vi "IMAQdx_grab_att.vi"() -> ()   [LabVIEW 2015]
doc: "The Grab VI acquires images continuously and displays the images in an image control using low-level acquisition VIs. A grab is appropriate for high-speed applications in which you need to process only one image at a time."
uses:
  <vilib>/vision/driver/IMAQdx.llb/IMAQdx Acquisition Mode.ctl
  <vilib>/vision/driver/IMAQdx.llb/IMAQdx Buffer Number Mode.ctl
  <vilib>/vision/driver/NI_Vision_Acquisition_Software.lvlib
  <resource>/objmgr/imaqdx.rc
  <vilib>/vision/NI_Vision_Development_Module.lvlib
panel:
  out "Luminance Plane":T1(plugin-control)
  out "Image":T1(plugin-control)
  out "ValueDBL 4":dbl
  out "MinDBL 5":dbl
  out "MaxDBL 5":dbl
  out "ActVal:Gain":string
  out "ValueU32 4":u32
  out "ValueDBL 3":dbl
  out "MinDBL 4":dbl
  out "MaxDBL 4":dbl
  out "ActGainMode":string
  out "ValueU32 3":u32
  out "ValueDBL 2":dbl
  out "MinDBL 3":dbl
  out "MaxDBL 3":dbl
  out "ActValue:Exposure":string
  out "ValueU32 2":u32
  out "ValueU32":u32
  out "ActExpMode":string
  out "MaxDBL 2":dbl
  out "MinDBL 2":dbl
  out "ValueDBL":dbl
  in  "Stop 4":bool
  out "Streaming Started":bool
  out "Stream completed":bool
  in  "Set: Exposure::Value":dbl=0.0625 caption="Exposure::Value" min=0.0 max=0.125
  in  "Gain::Mode":u32(ring)=2 caption="Exposure::Mode" items=["Auto"=1, "Manual"=2]
  in  "Exposure::Mode":u32(ring)=2 items=["Auto"=1, "Manual"=2]
  in  "Set Gain":bool
  in  "Set Exposure":bool
  in  "Stop 3":bool
  out "output cluster":cluster{sgl, sgl}
  out "Last Mouse Position:All Elements":cluster{"X":i32, "Y":i32}
  in  "Set: Gain::Value":i64 caption="Gain::Value" min=0 max=1728 step=1
  in  "Pixel Distances":T2={"X Step"=5.2, "Y Step"=5.2, "Unit"=enum."Micrometer"} {"Y Step" format="%.2f"; "X Step" format="%.2f"}
  out "error out":errorcluster
  in  "Camera Name":refnum<k21>="cam0" caption="IMAQdx Session"
  out "Buffer Number":u32
  out "Frame Rate":dbl(knob) scale=0.0..20.0
  in  "Stop":bool
  # "Overview: Demonstrates how to acquire continuous images from a camera using low level acquisition functions.\nRequirements: Vision Acquisition Software\nInstructions:\n1. Select the Camera Name\n2. Run the VI"
  # "x /µm"
  # "y /µm"
  # "ExpMode"
  # "ExpVal"
  # "GainMode"
  # "GainValue"
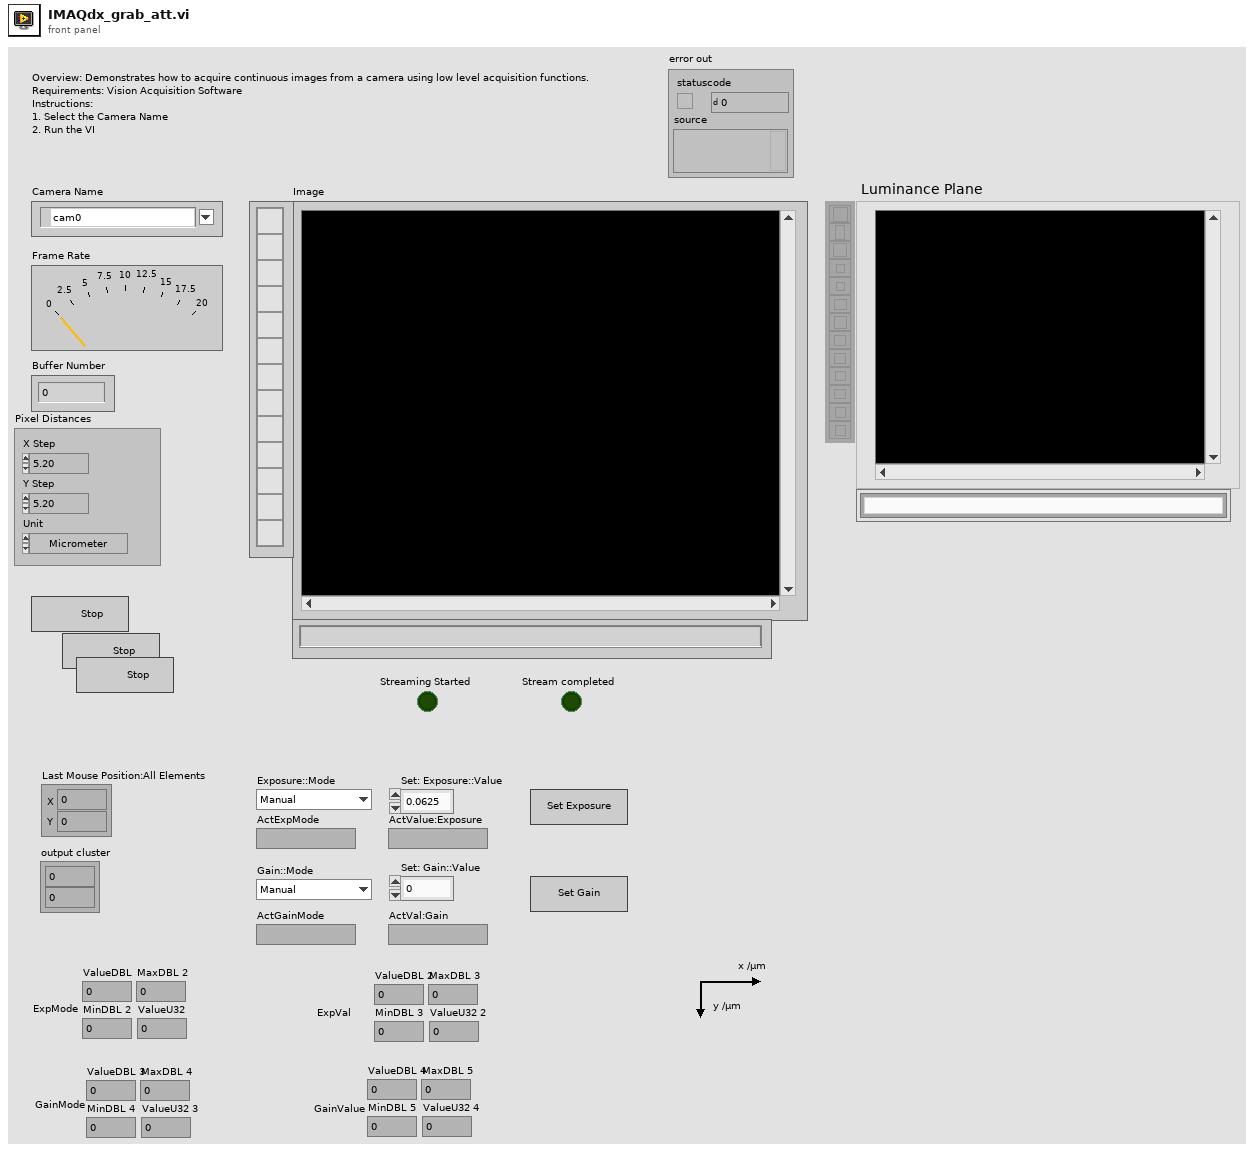
[diagram p1: front panel]
types:
  T1 = typedef "IMAQ Image.ctl" = refnum<image>
  T2 = typedef "Simple Grid Descriptor" = cluster{"X Step":sgl, "Y Step":sgl, "Unit":T3}
  T3 = typedef "Image Unit" = enum32{"Undefined", "Angström", "Micrometer", "Millimeter", "Centimeter", "Meter", "Kilometer", "Microinch", "Inch", "Feet", "Nautical miles", "Standard miles", "Steps"}
  T4 = typedef "Image Type" = u32
  T5 = typedef "NI_Vision_Acquisition_Software.lvlib/IMAQdx Acquisition Mode.ctl" = enum32{"One Shot", "Continuous"}
  T6 = typedef "IMAQdx.ctl" = refnum<k21>
  T7 = enum8{"Enabled", "Disabled", "Disabled and Grayed Out"}
  T8 = typedef "NI_Vision_Acquisition_Software.lvlib/IMAQdx Buffer Number Mode.ctl" = enum32{"Next", "Last", "Buffer Number", "Every", "Last New"}
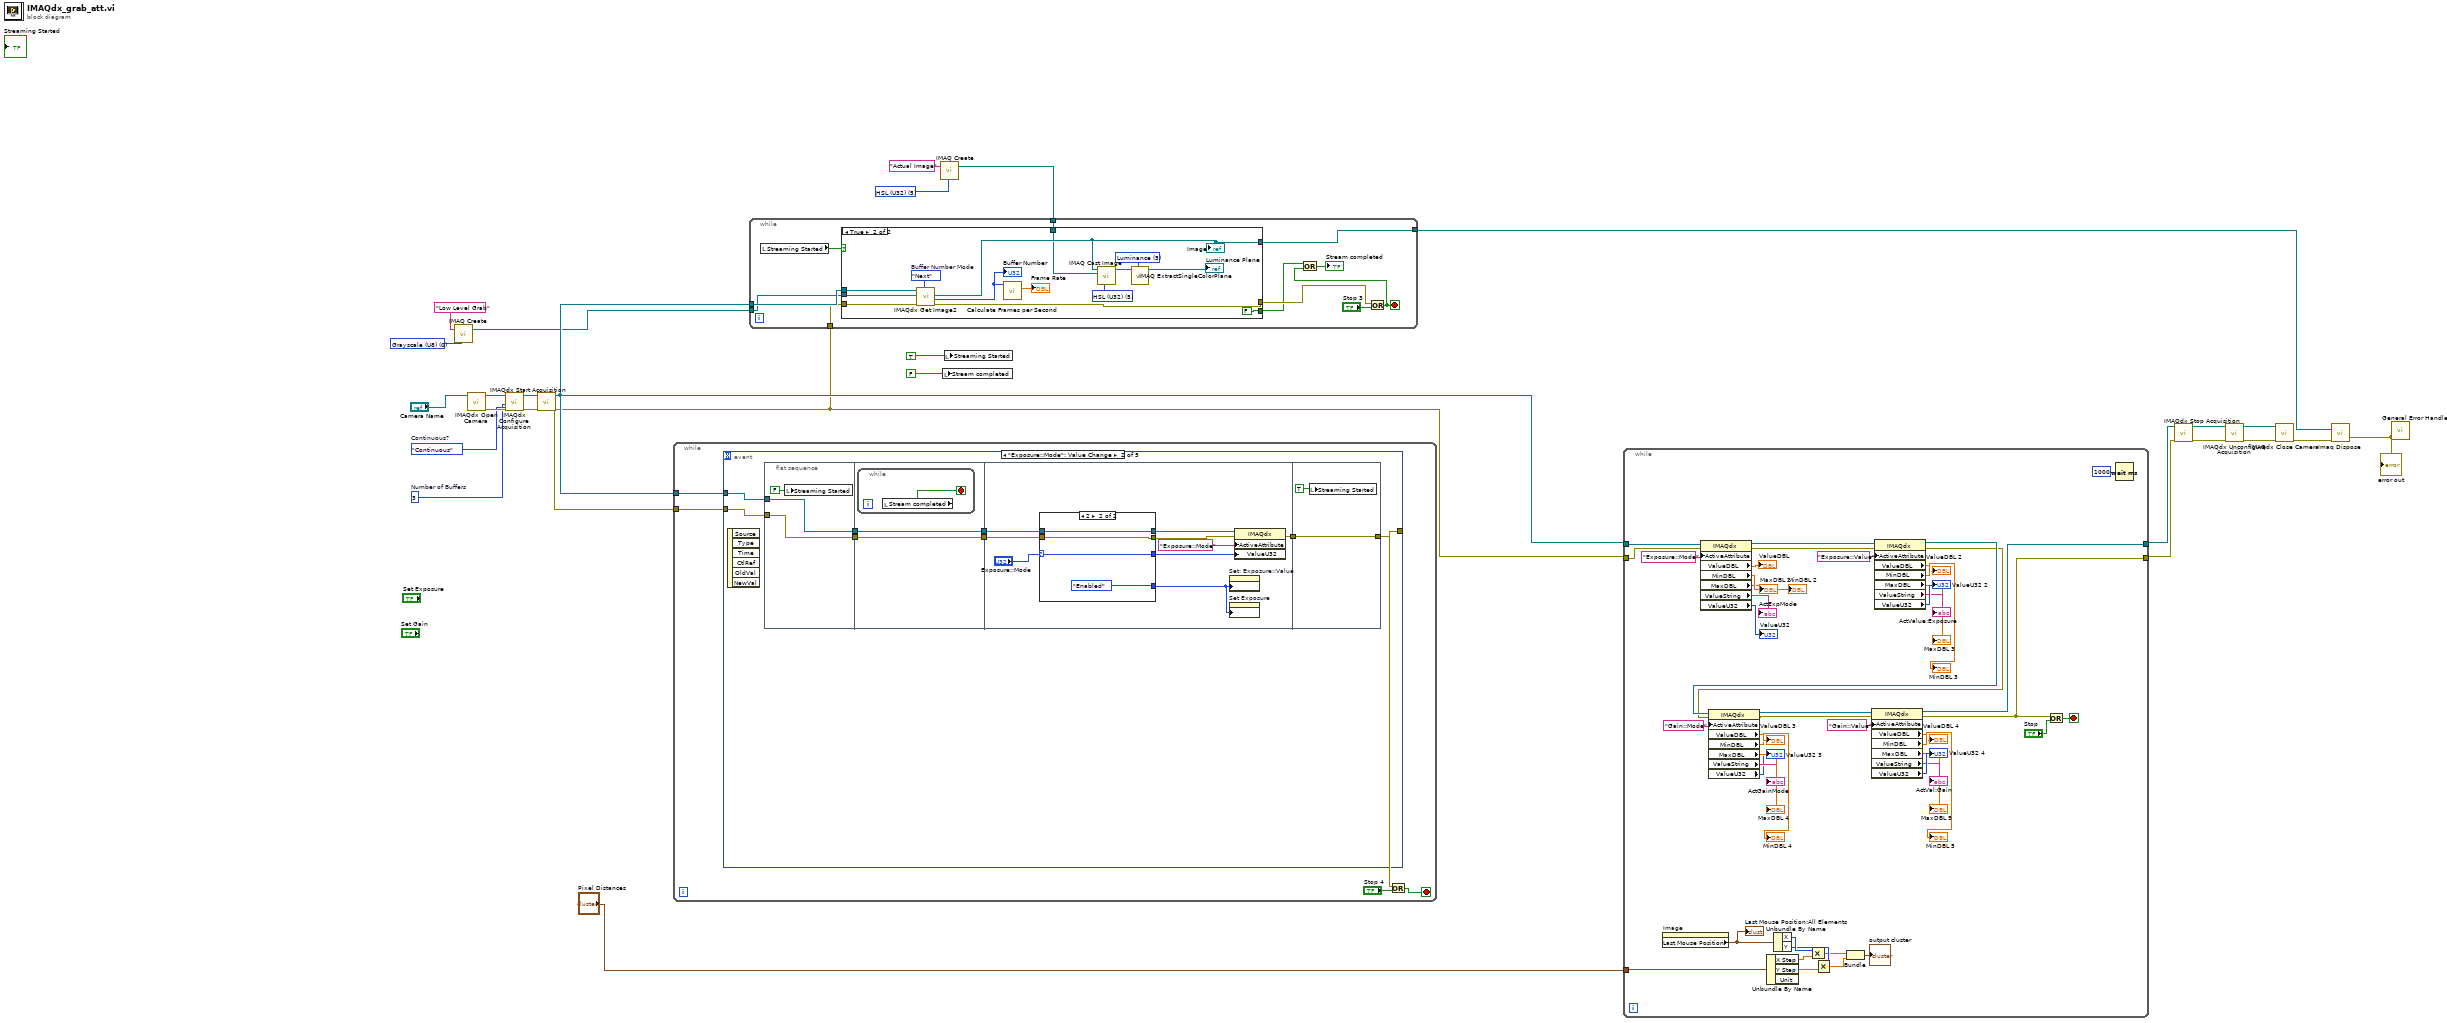
[diagram p0: block diagram]
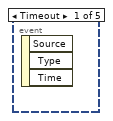
[diagram p2: hidden frame]
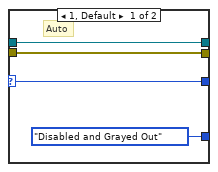
[diagram p3: hidden frame]
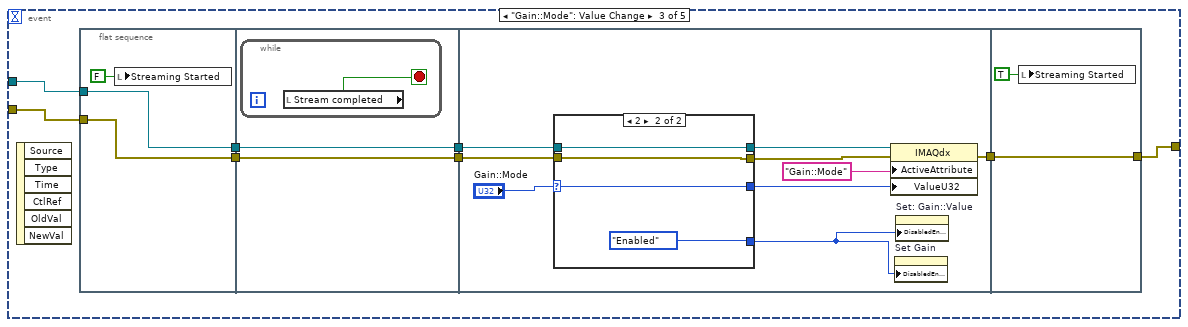
[diagram p4: hidden frame]
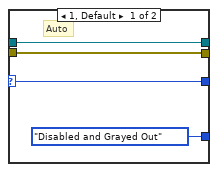
[diagram p5: hidden frame]
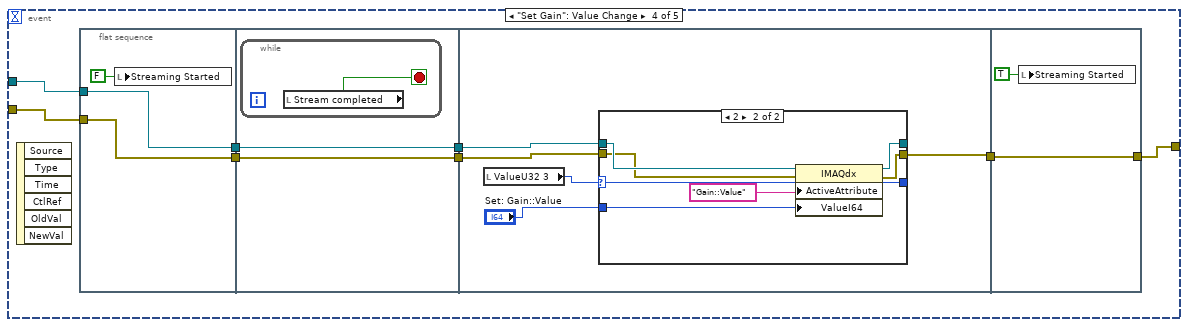
[diagram p6: hidden frame]
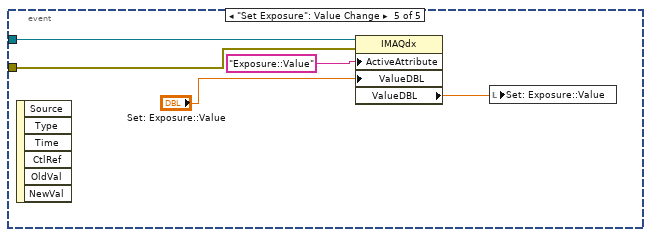
[diagram p8: hidden frame]
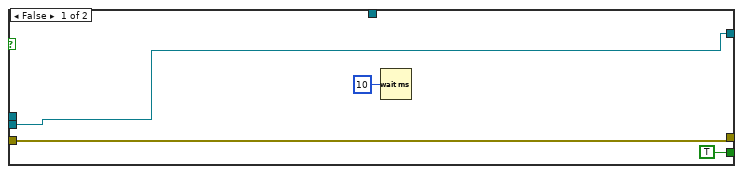
[diagram p9: hidden frame]
diagram:
  w2 = T4 5 items=["Grayscale (U8)", "Grayscale (I16)", "Grayscale (SGL)", "Complex (CSG)", "RGB (U32)", "HSL (U32)", "RGB (U64)", "Grayscale (U16)"] ("Image Type")
  w17 = T4 0 items=["Grayscale (U8)", "Grayscale (I16)", "Grayscale (SGL)", "Complex (CSG)", "RGB (U32)", "HSL (U32)", "RGB (U64)", "Grayscale (U16)"] ("Image Type")
  w24 = u32 3  # Number of Buffers
  w25 = IMAQdx_Acquisition_Mode."Continuous"  # Continuous?
  n1 = call "IMAQ Create"("Image Name"="Low Level Grab", "Image Type"=w17) -> ("New Image"=w9:T1)  [unwired: 2 in, 2 out]
  n2 = call <vilib>:"IMAQdx Open Camera.vi"("Session In"="Camera Name") -> ("error out"=w26:errorcluster, "Session Out"=w18:T6)  [unwired: 2 in, 7 out]
  n3 = call <vilib>:"IMAQdx Configure Acquisition.vi"("error in"=w26, "Number of Buffers"=w24, "Continuous?"=w25, "Session In"=w18) -> ("error out"=w16:errorcluster, "Session Out"=w12:T6)  [unwired: 6 out]
  n4 = call <vilib>:"IMAQdx Start Acquisition.vi"("error in"=w16, "Session In"=w12) -> ("error out"=w7:errorcluster, "Session Out"=w10:T6)  [unwired: 8 out]
  n5 = while {
    tunnel: w10 -> [w32]
    tunnel: w7 -> [w31]
    stop <- w29 stop-if-true
    n6 = event shown="[1] \"Exposure::Mode\": Value Change" {
      selector: _ -> [_ _ _ _ _]
      dyn-events: _ -> [_ _ _ _ _]
      timeout: _ -> [_ _ _ _ _]
      tunnel: w32 -> [_ w40 w73 w106 w133]
      tunnel: w31 -> [_ w37 w70 w103 w132]
      tunnel: [_ w34 w67 w100 _] -> w28
      event Timeout {
        n7 = event-data() -> ()  [unwired: 1 in, 3 out]
      }
      event "Exposure::Mode": Value Change {
        n8 = event-data() -> ()  [unwired: 1 in, 6 out]
        n9 = flat-sequence {
          tunnel: w40 -> [w42]
          tunnel: [w42] -> w39
          tunnel: w37 -> [w41]
          tunnel: [w41] -> w36
          tunnel: w39 -> [w45]
          tunnel: [w45] -> w38
          tunnel: w36 -> [w44]
          tunnel: [w44] -> w35
          tunnel: w38 -> [w54]
          tunnel: w35 -> [w53]
          tunnel: [w48] -> w33
          tunnel: [w65] -> w34
          tunnel: w33 -> [w65]
          frame #0 {
            n10 = local write "Streaming Started"(FALSE ("Streaming Started")) -> ()
          }
          frame #1 {
            n11 = while {
              stop <- w46 stop-if-true
              n12 = local read "Stream completed"() -> (w46:bool)
            }
          }
          frame #2 {
            n13 = case shown="2" "Exposure::Mode" {
              selector: "Exposure::Mode" -> [w57 w60]
              tunnel: w54 -> [w59 w62]
              tunnel: w53 -> [w58 w61]
              tunnel: [w59 w62] -> w52
              tunnel: [w58 w61] -> w51
              tunnel: [w57 w60] -> w50
              tunnel: [T7."Disabled and Grayed Out" ("Disabled") T7."Enabled" ("Disabled")] -> w47
              frame 1, Default {
                # "Auto"
              }
              frame 2 {
              }
            }
            n14 = property on="Set: Exposure::Value" class="DigNum (strict)"("DisabledEnum"=w47) -> ()  [unwired: 2 in, 2 out]
            n15 = property on="Set Exposure" class="Bool"("DisabledEnum"=w47) -> ()  [unwired: 2 in, 2 out]
            n16 = property class="IMAQdx"(reference=w52, error in=w51, "ActiveAttribute"="Exposure::Mode", "ValueU32"=w50) -> (error out=w48:errorcluster)  [unwired: 1 out]
          }
          frame #3 {
            n17 = local write "Streaming Started"(TRUE ("Streaming Started")) -> ()
          }
        }
      }
      event "Gain::Mode": Value Change {
        n18 = event-data() -> ()  [unwired: 1 in, 6 out]
        n19 = flat-sequence {
          tunnel: w73 -> [w75]
          tunnel: [w75] -> w72
          tunnel: w70 -> [w74]
          tunnel: [w74] -> w69
          tunnel: w72 -> [w78]
          tunnel: [w78] -> w71
          tunnel: w69 -> [w77]
          tunnel: [w77] -> w68
          tunnel: w71 -> [w88]
          tunnel: w68 -> [w87]
          tunnel: [w82] -> w66
          tunnel: [w98] -> w67
          tunnel: w66 -> [w98]
          frame #0 {
            n20 = local write "Streaming Started"(FALSE ("Streaming Started")) -> ()
          }
          frame #1 {
            n21 = while {
              stop <- w79 stop-if-true
              n22 = local read "Stream completed"() -> (w79:bool)
            }
          }
          frame #2 {
            n23 = case shown="2" "Gain::Mode" {
              selector: "Gain::Mode" -> [w90 w93]
              tunnel: w88 -> [w92 w95]
              tunnel: w87 -> [w91 w94]
              tunnel: [w92 w95] -> w86
              tunnel: [w91 w94] -> w85
              tunnel: [w90 w93] -> w84
              tunnel: [T7."Disabled and Grayed Out" ("Disabled") T7."Enabled" ("Disabled")] -> w80
              frame 1, Default {
                # "Auto"
              }
              frame 2 {
              }
            }
            n24 = property class="IMAQdx"(reference=w86, error in=w85, "ActiveAttribute"="Gain::Mode", "ValueU32"=w84) -> (error out=w82:errorcluster)  [unwired: 1 out]
            n25 = property on="Set Gain" class="Bool"("DisabledEnum"=w80) -> ()  [unwired: 2 in, 2 out]
            n26 = property on="Set: Gain::Value" class="DigNum (strict)"("DisabledEnum"=w80) -> ()  [unwired: 2 in, 2 out]
          }
          frame #3 {
            n27 = local write "Streaming Started"(TRUE ("Streaming Started")) -> ()
          }
        }
      }
      event "Set Gain": Value Change {
        n28 = event-data() -> ()  [unwired: 1 in, 6 out]
        n29 = flat-sequence {
          tunnel: w106 -> [w108]
          tunnel: [w108] -> w105
          tunnel: w103 -> [w107]
          tunnel: [w107] -> w102
          tunnel: w105 -> [w111]
          tunnel: [w111] -> w104
          tunnel: w102 -> [w110]
          tunnel: [w110] -> w101
          tunnel: w104 -> [w117]
          tunnel: w101 -> [w116]
          tunnel: [w115] -> w99
          tunnel: [w129] -> w100
          tunnel: w99 -> [w129]
          frame #0 {
            n30 = local write "Streaming Started"(FALSE ("Streaming Started")) -> ()
          }
          frame #1 {
            n31 = while {
              stop <- w112 stop-if-true
              n32 = local read "Stream completed"() -> (w112:bool)
            }
          }
          frame #2 {
            n33 = local read "ValueU32 3"() -> (w114:u32)
            n34 = case shown="2" w114 {
              selector: w114 -> [w118 w127]
              tunnel: w117 -> [w120 w125]
              tunnel: w116 -> [w119 w124]
              tunnel: [w120 w122] -> _
              tunnel: [w119 w121] -> w115
              tunnel: [w118 w127] -> _
              tunnel: "Set: Gain::Value" -> [_ w123]
              frame 1, Default {
                # "Auto"
              }
              frame 2 {
                n35 = property class="IMAQdx"(reference=w125, error in=w124, "ActiveAttribute"="Gain::Value", "ValueI64"=w123) -> (reference out=w122:T6, error out=w121:errorcluster)
              }
            }
          }
          frame #3 {
            n36 = local write "Streaming Started"(TRUE ("Streaming Started")) -> ()
          }
        }
      }
      event "Set Exposure": Value Change {
        n37 = event-data() -> ()  [unwired: 1 in, 6 out]
        n38 = property class="IMAQdx"(reference=w133, error in=w132, "ActiveAttribute"="Exposure::Value", "ValueDBL"="Set: Exposure::Value") -> ("ValueDBL"=w130:dbl)  [unwired: 2 out]
        n39 = local write "Set: Exposure::Value"(w130) -> ()
      }
    }
    n40 = Or(x=w28, y="Stop 4") -> (x .or. y?=w29:bool)
  }
  n41 = call "IMAQ Create"("Image Name"="Actual Image", "Image Type"=w2) -> ("New Image"=w1:T1)  [unwired: 3 in, 1 out]
  n42 = while {
    tunnel: [w144] -> w11
    tunnel: w10 -> [w145]
    tunnel: w9 -> [w139]
    tunnel: w7 -> [w143]
    tunnel: w1 -> [w135]
    stop <- w136 stop-if-true
    n43 = local read "Streaming Started"() -> (w142:bool)
    n44 = case shown="True" w142 {
      tunnel: w145 -> [_ w160]
      tunnel: [w146 w151] -> w144
      tunnel: w139 -> [w146 w159]
      tunnel: w143 -> [w147 w158]
      tunnel: [TRUE ("Set Attribute") FALSE ("Set Attribute")] -> w137
      tunnel: [w147 w156] -> w140
      tunnel: w135 -> [_ w150]
      frame False {
        n45 = Wait (ms)(milliseconds to wait=u32 10) -> ()  [unwired: 1 out]
      }
      frame True {
        w154 = 5 items=["Red", "Green", "Blue", "Hue", "Saturation", "Luminance", "Value", "Intensity"] ("Color Plane")
        w155 = T4 5 items=["Grayscale (U8)", "Grayscale (I16)", "Grayscale (SGL)", "Complex (CSG)", "RGB (U32)", "HSL (U32)", "RGB (U64)"] ("Image Type")
        w162 = IMAQdx_Buffer_Number_Mode."Next"  # Buffer Number Mode
        n46 = call <vilib>:"IMAQdx Get Image2.vi"("Buffer Number Mode (Next)"=w162, "error in"=w158, "Image In"=w159, "Session In"=w160) -> ("error out"=w156:errorcluster, "Buffer Number Out"=w163:u32, "Image Out"=w151:T1)  [unwired: 4 in, 1 out]
        "Buffer Number" <- w163
        "Image" <- w151
        n47 = call <vilib>:"Calculate Frames per Second.vi"("Buffer Number"=w163) -> ("Processed Frames/s"=→"Frame Rate":dbl)  [unwired: 8 in, 2 out]
        n48 = call "IMAQ Cast Image"("Image Type"=w155, "Image Dst"=w150, "Image Src"=w151) -> ("Image Dst Out"=w153:T1)  [unwired: 7 in, 1 out]
        n49 = call "IMAQ ExtractSingleColorPlane"("Color Plane"=w154, "Image Src"=w153) -> ("Image Dst Out"=→"Luminance Plane":T1)  [unwired: 8 in, 1 out]
      }
    }
    n50 = Or(x=w140, y="Stop 3") -> (x .or. y?=w136:bool)
    n51 = Or(x=w137, y=w136) -> (x .or. y?=→"Stream completed":bool)
  }
  n52 = local write "Stream completed"(FALSE ("Streaming Started")) -> ()
  n53 = local write "Streaming Started"(TRUE ("Streaming Started")) -> ()
  n54 = while {
    tunnel: [w166] -> w8
    tunnel: w7 -> [w197]
    tunnel: w10 -> [w198]
    tunnel: [w165] -> w15
    tunnel: "Pixel Distances" -> [w207]
    stop <- w209 stop-if-true
    n55 = property on="Image" class="ImageControl"() -> ("Last Mouse Position"=w164:cluster{"X":i32, "Y":i32})  [unwired: 2 in, 2 out]
    "Last Mouse Position:All Elements" <- w164
    n56 = property class="IMAQdx"(reference=w198, error in=w197, "ActiveAttribute"="Exposure::Mode") -> (reference out=w172:T6, error out=w171:errorcluster, "ValueDBL"=→"ValueDBL":dbl, "MinDBL"=→"MinDBL 2":dbl, "MaxDBL"=→"MaxDBL 2":dbl, "ValueString"=→"ActExpMode":string, "ValueU32"=→"ValueU32":u32)
    n57 = Unbundle By Name(w207) -> ("X Step"=w205:sgl, "Y Step"=w203:sgl)  [unwired: 1 out]
    n58 = Unbundle By Name(w164) -> ("X"=w206:i32, "Y"=w204:i32)
    n59 = Multiply(x=w206, y=w205) -> (x*y=w201:sgl)
    n60 = Multiply(x=w204, y=w203) -> (x*y=w202:sgl)
    n61 = Bundle(w201, w202) -> (→"output cluster":cluster{sgl, sgl})  [unwired: 1 in]
    n62 = property class="IMAQdx"(reference=w172, error in=w171, "ActiveAttribute"="Exposure::Value") -> (reference out=w170:T6, error out=w169:errorcluster, "ValueDBL"=→"ValueDBL 2":dbl, "MinDBL"=→"MinDBL 3":dbl, "MaxDBL"=→"MaxDBL 3":dbl, "ValueString"=→"ActValue:Exposure":string, "ValueU32"=→"ValueU32 2":u32)
    n63 = property class="IMAQdx"(reference=w170, error in=w169, "ActiveAttribute"="Gain::Mode") -> (reference out=w168:T6, error out=w167:errorcluster, "ValueDBL"=→"ValueDBL 3":dbl, "MinDBL"=→"MinDBL 4":dbl, "MaxDBL"=→"MaxDBL 4":dbl, "ValueString"=→"ActGainMode":string, "ValueU32"=→"ValueU32 3":u32)
    n64 = property class="IMAQdx"(reference=w168, error in=w167, "ActiveAttribute"="Gain::Value") -> (reference out=w166:T6, error out=w165:errorcluster, "ValueDBL"=→"ValueDBL 4":dbl, "MinDBL"=→"MinDBL 5":dbl, "MaxDBL"=→"MaxDBL 5":dbl, "ValueString"=→"ActVal:Gain":string, "ValueU32"=→"ValueU32 4":u32)
    n65 = Or(x=w165, y="Stop") -> (x .or. y?=w209:bool)
    n66 = Wait (ms)(milliseconds to wait=u32 1000) -> ()  [unwired: 1 out]
  }
  n67 = call <vilib>:"IMAQdx Stop Acquisition.vi"("error in"=w15, "Session In"=w8) -> ("error out"=w13:errorcluster, "Session Out"=w14:T6)  [unwired: 8 out]
  n68 = call <vilib>:"IMAQdx Unconfigure Acquisition.vi"("error in"=w13, "Session In"=w14) -> ("error out"=w23:errorcluster, "Session Out"=w22:T6)  [unwired: 8 out]
  n69 = call <vilib>:"IMAQdx Close Camera.vi"("error in"=w23, "Session In"=w22) -> ("error out"=w21:errorcluster)  [unwired: 9 out]
  n70 = call "Imaq Dispose"("Image"=w11, "error in (no error)"=w21) -> ("error out"=w20:errorcluster)  [unwired: 4 in]
  "error out" <- w20
  n71 = call <vilib>:"General Error Handler.vi"("error in (no error)"=w20) -> ()  [unwired: 2 in, 13 out]
